vi "Funktionen Automatisch beenden.vi"(9 "Zeit":sgl, 11 "ausgewählte Funktion":T1) -> (1 "Zeit":sgl)   [LabVIEW 2020, in "Funktionstasten.lvlib"]
uses:
  Funktionstasten.lvlib
  Zustaende.ctl
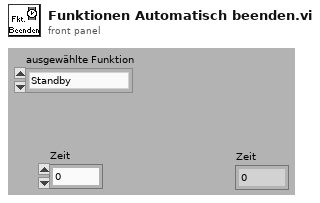
[diagram p1: front panel]
types:
  T1 = typedef "Funktionstasten.lvlib/Zustaende.ctl" = enum16{"Standby", "Pause", "Eco", "Messen", "Kalibrieren", "Spülen Filter", "Spülen Leitung", "Umgebungsluft", "0-Gas", "Cal-Gas", "CG zu PNS", "-------------", "Init 1", "Init 2", "Init 3", "Init 4", "Messen vorbereiten", "Messen durchführen", "Exit"}
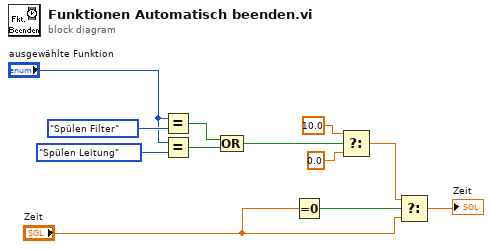
[diagram p0: block diagram]
diagram:
  n1 = Equal?(x="ausgewählte Funktion", y=Zustaende."Spülen Filter") -> (x = y?=w9:bool)
  n2 = Equal?(x="ausgewählte Funktion", y=Zustaende."Spülen Leitung") -> (x = y?=w8:bool)
  n3 = Compound Arithmetic op=OR(w9, w8) -> (w7:bool)
  n4 = Equal To 0?(x="Zeit") -> (x = 0?=w4:bool)
  n5 = Select(t=sgl 10.0, s=w7, f=sgl 0.0) -> (s? t:f=w3:sgl)
  n6 = Select(t=w3, s=w4, f="Zeit") -> (s? t:f=→"Zeit":sgl)
